vi "count targets.vi"() -> (3 "target type count":i32)   [LabVIEW 2013, in "TBM configuration.lvclass"]
doc: "A helper which indicates the quantity of targets supported by the framework."
uses:
  TBM configuration.lvclass
  Target Types.ctl
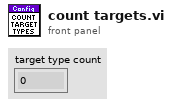
[diagram p1: front panel]
types:
  T1 = typedef "TBM configuration.lvclass/Target Types.ctl" = enum16{"Windows", "Mac", "Linux", "Linux RT ARM", "VxWorks", "Pharlap", "Other", "Linux RT x64"}
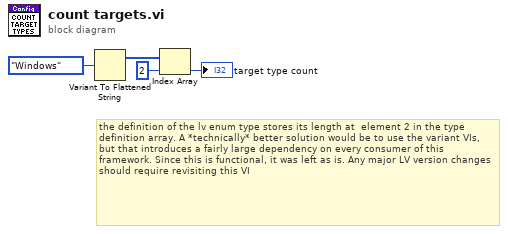
[diagram p0: block diagram]
diagram:
  # "the definition of the lv enum type stores its length at  element 2 in the type definition array. A *technically* better solution would be to use the variant VIs, but that introduces a fairly large dependency on every consumer of this framework. Since this is functional, it was left as is. Any major LV version changes should require revisiting this VI"
  n1 = Variant To Flattened String(Variant=Target_Types."Windows" ("Target Types")) -> (1:w3:i16[])  [unwired: 1 out]
  n2 = Index Array(array=w3, index=2) -> (element=→"target type count":i16)
